vi "SHA-1 Test.vi"() -> ()   [LabVIEW 2014]
panel:
  out "SHA512  length":i32=128
  in  "SHA512":string="96f06aec039a44b9b053079476554fd6954ecd5a126692463cc3dab112b172199a3ea8a32ab998156ec47157b1bb595d3aa88277a89cb2a78302668d8560d50e"
  out "SHA1 length":i32=40
  out "MD5 length":i32=32
  out "MD5 message-digest":string="6746b644f1a32176428df54bc8c6bbfd"
  in  "Message String":string="vctAdmin"
  out "SHA1 string":string="442A0DBBB90711CFDFC0E47CD80FF5F67928C03D"
  out "SHA1 Data":u8[](array[numeric])=[68, 42, 13, 187, 185, 7, 17, 207, 223, 192, 228, 124, 216, 15, 245, 246, 121, 40, 192, 61] format="%.0x"
  # "SHA1(\"\")\n = da39a3ee 5e6b4b0d 3255bfef 95601890 afd80709"
  # "SHA1(\"The quick brown fox jumps over the lazy dog\") \n = 2fd4e1c6 7a2d28fc ed849ee1 bb76e739 1b93eb12"
  # "minor change - dog -> cog (notice large change, aka avalache effect, in digest)"
  # "SHA1(\"The quick brown fox jumps over the lazy cog\") \n = de9f2c7f d25e1b3a fad3e85a 0bd17d9b 100db4b3"
  # "442A0DBBB90711CFDFC0E47CD80FF5F67928C03D"
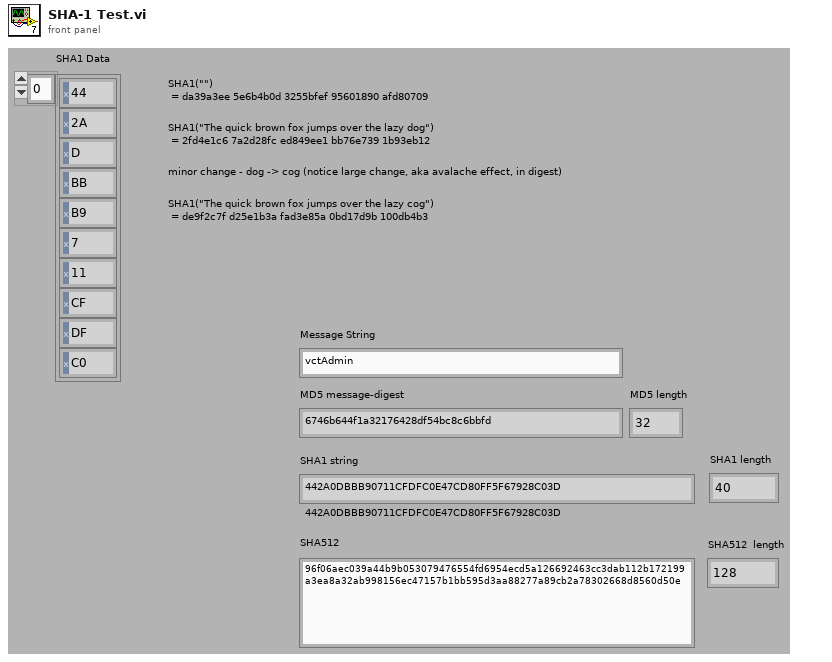
[diagram p1: front panel]
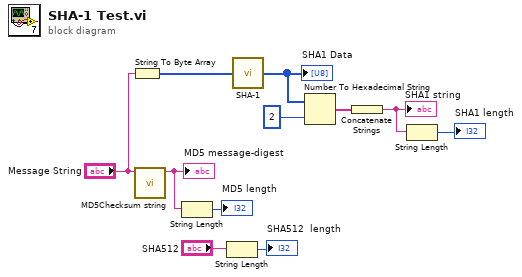
[diagram p0: block diagram]
diagram:
  n1 = String To Byte Array(string="Message String") -> (unsigned byte array=w11:u8[])
  n2 = call <vilib>:"MD5Checksum string.vi"("Message String"="Message String") -> ("MD5 message-digest"=w10:string)  [unwired: 10 in]
  "MD5 message-digest" <- w10
  n3 = String Length(string=w10) -> (length=→"MD5 length":i32)
  n4 = String Length(string="SHA512") -> (length=→"SHA512  length":i32)
  n5 = call "SHA-1.vi"("Data"=w11) -> ("message-digest"=w7:u8[])
  "SHA1 Data" <- w7
  n6 = Number To Hexadecimal String(1:i16 2 ("width (-)"), 2:w7) -> (0:w5:string[])
  n7 = Concatenate Strings(w5) -> (w4:string)
  "SHA1 string" <- w4
  n8 = String Length(string=w4) -> (length=→"SHA1 length":i32)
